vi "Increment Program Counter.vi"(8 "error in (no error)":errorcluster, 11 "TD4 in":refnum<class "TD4.lvclass">) -> (0 "error out":errorcluster, 3 "TD4 out":refnum<class "TD4.lvclass">)   [LabVIEW 2025, in "TD4.lvclass"]
uses:
  TD4.lvclass
  TD4.lvclass/TD4.ctl
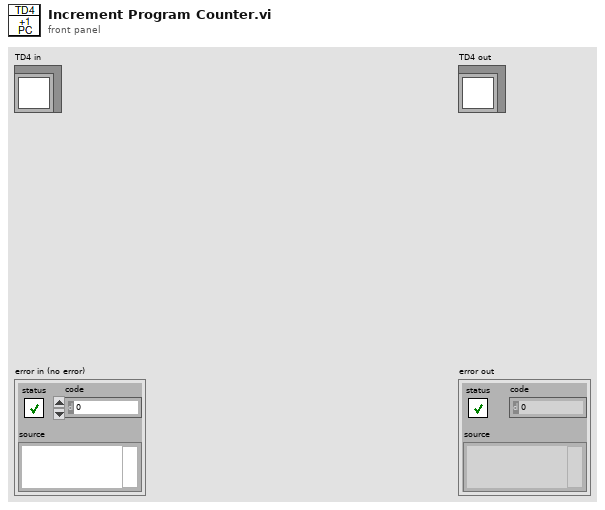
[diagram p1: front panel]
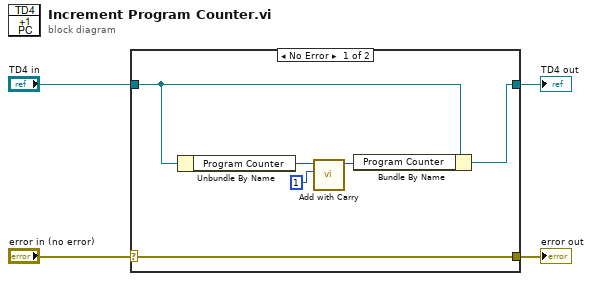
[diagram p0: block diagram]
diagram:
  n1 = case shown="No Error" "error in (no error)" {
    selector: "error in (no error)" -> [w10 w11]
    tunnel: [w10 w11] -> w3
    tunnel: [w9 w12] -> w1
    tunnel: "TD4 in" -> [w8 w12]
    frame No Error {
      n2 = Unbundle By Name(w8) -> ("Program Counter"=w7:u8)
      n3 = call "Add with Carry.vi"("Input 2"=u8 1, "Input 1"=w7) -> ("Output"=w5:u8)  [unwired: 8 in, 1 out]
      n4 = Bundle By Name(cluster=w8, "Program Counter"=w5) -> (w9:refnum<class "TD4.lvclass">)
    }
    frame Error {
    }
  }
  "error out" <- w3
  "TD4 out" <- w1
